vi "Create Data Container.vi"(8 "error in (no error)":errorcluster, 10 "TaskName":string, 11 "DAQ_Module in":refnum<class "DAQ_Module.lvclass">) -> (0 "error out":errorcluster, 2 "Container":refnum<data-value>, 3 "DAQ_Module out":refnum<class "DAQ_Module.lvclass">)   [LabVIEW 2025, in "DAQ_Module.lvlib" / "DAQ_Module.lvclass"]
uses:
  DAQ_Module.lvclass
  DAQ_Abstr/Task_Abstr/Task_Abstr/DataContainer.ctl
  DAQ_Abstr/Task_Abstr/Task_Abstr/WaveformData.ctl
  DAQ_Module.lvclass/DAQ_Module.ctl
  DAQ_Abstr/Task_Abstr/Task_Abstr/Task_Abstr.lvclass
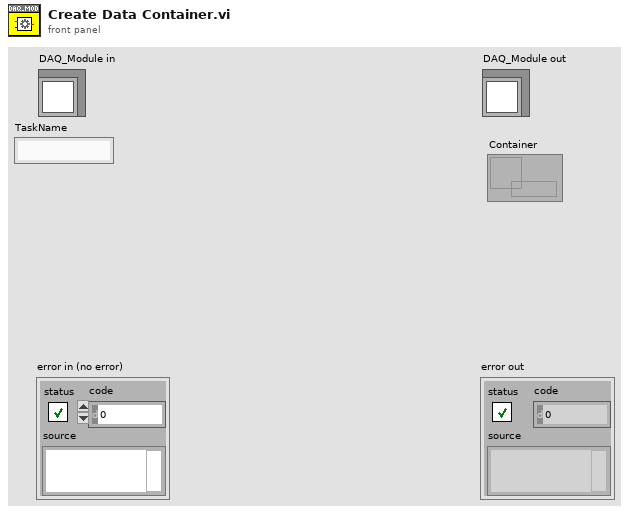
[diagram p1: front panel]
types:
  T1 = typedef "Task_Abstr.lvlib/Task_Abstr.lvclass/DataContainer.ctl" = map{string, T2}
  T2 = typedef "Task_Abstr.lvlib/Task_Abstr.lvclass/WaveformData.ctl" = cluster{"StartTime":timestamp, "StopTime":timestamp, "Waveform":waveform(dbl)[]}
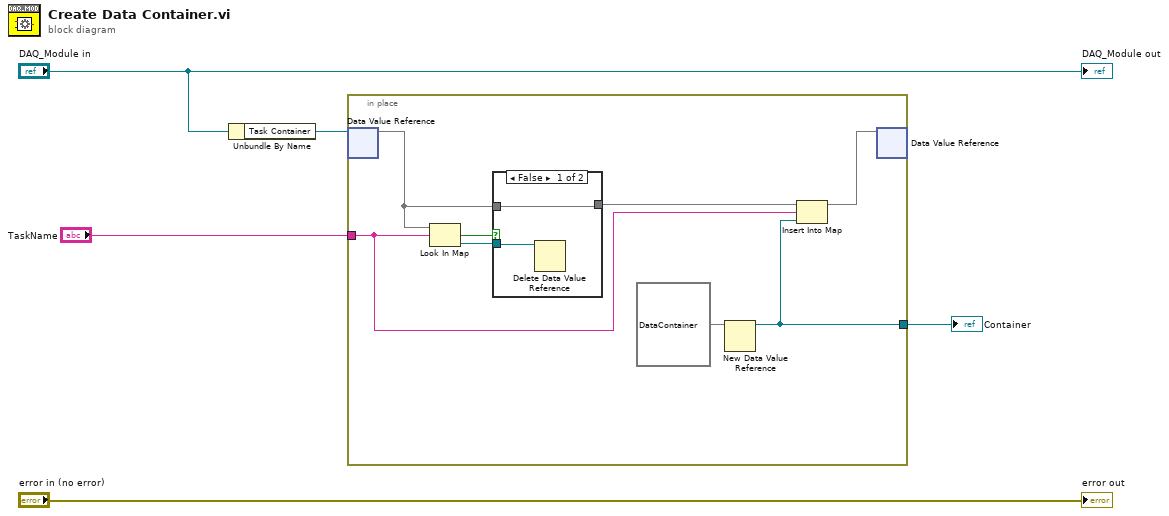
[diagram p0: block diagram]
diagram:
  n1 = Unbundle By Name("DAQ_Module in") -> ("Task Container"=w2:refnum<data-value>)
  n2 = in-place {
    in-place-border: "TaskName" -> [w8]
    in-place-border: [w6] -> w1
    n3 = in-place-dvr #1(w2) -> (w12:map{string, refnum<data-value>})  [unwired: 1 out]
    n4 = Look In Map(map=w12, key=w8) -> (key not found?=w13:bool, value=w11:refnum<data-value>)  [unwired: 1 in]
    n5 = case shown="False" w13 {
      tunnel: w12 -> [w14 w16]
      tunnel: [w14 w16] -> w9
      tunnel: w11 -> [w15 _]
      frame False {
        n6 = Delete Data Value Reference(data value reference=w15) -> ()  [unwired: 1 in, 2 out]
      }
      frame True {
      }
    }
    n7 = New Data Value Reference(data value=T1 {} ("map")) -> (data value reference=w6:refnum<data-value>)  [unwired: 1 in, 1 out]
    n8 = Insert Into Map(map in=w9, key=w8, value=w6) -> (map out=w7:map{string, refnum<data-value>})  [unwired: 2 out]
    n9 = in-place-dvr #1(w7) -> ()  [unwired: 2 out]
  }
  "Container" <- w1
  "error out" <- "error in (no error)"
  "DAQ_Module out" <- "DAQ_Module in"
